vi "Get value OUT2.vi"(0 "Keyence":T2={"Serial port sem"=refnum, "Serial port handle"="", "Baud rate"=9600}, 5 "error in":errorcluster) -> (11 "Start transfer":u32, 14 "Keyence out":T2={"Serial port sem"=refnum, "Serial port handle"="", "Baud rate"=9600}, 16 "Distances":dbl[](array[numeric]), 17 "Distance":dbl, 19 "error out":errorcluster)   [LabVIEW 2018]
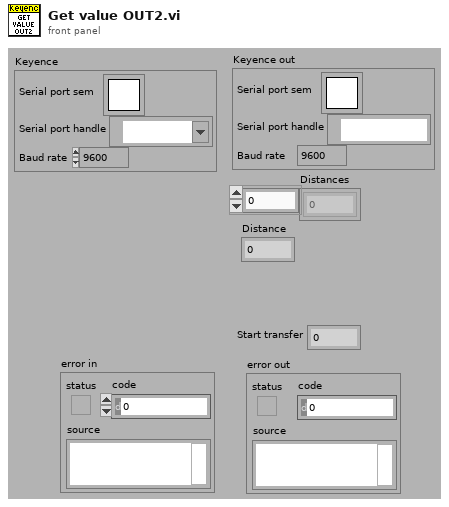
[diagram p1: front panel]
types:
  T1 = typedef "Semaphore RefNum" = refnum<k1>
  T2 = cluster{"Serial port sem":T1, "Serial port handle":refnum<visa-resource-name>, "Baud rate":u32}
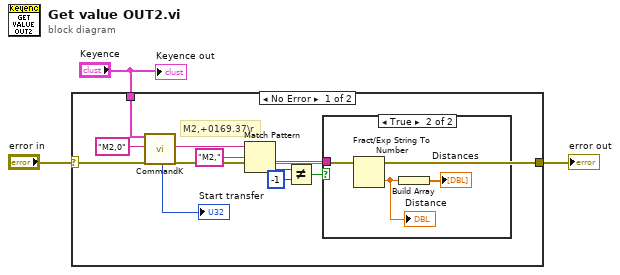
[diagram p0: block diagram]
diagram:
  n1 = case shown="No Error" "error in" {
    selector: "error in" -> [w14 w18]
    tunnel: [w6 w18] -> w3
    tunnel: "Keyence" -> [w5 _]
    frame No Error {
      # "M2,+0169.37\\r"
      n2 = call "CommandK.vi"("Keyence"=w5, "Command"="M2,0", "error in"=w14) -> ("Command time, ms"=→"Start transfer":u32, "Answer"=w11:string, "error out"=w6:errorcluster)  [unwired: 13 in, 1 out]
      n3 = Match Pattern(string=w11, regular expression="M2," ("string")) -> (after substring=w10:string, offset past match=w9:i32)  [unwired: 1 in, 2 out]
      n4 = Not Equal?(x=w9, y=-1) -> (x != y?=w7:bool)
      n5 = case shown="True" w7 {
        tunnel: w10 -> [_ w17]
        frame False {
        }
        frame True {
          n6 = Fract/Exp String To Number(string=w17) -> (number=w16:dbl)  [unwired: 3 in, 1 out]
          "Distance" <- w16
          n7 = Build Array(w16) -> (→"Distances":dbl[])
        }
      }
    }
    frame Error {
    }
  }
  "error out" <- w3
  "Keyence out" <- "Keyence"
